vi "Full Icon Size.vi"(8 "error in":errorcluster, 11 "VI in":refnum<vi>) -> (0 "error out":errorcluster, 3 "Full Icon Size?":bool)   [LabVIEW 2024]
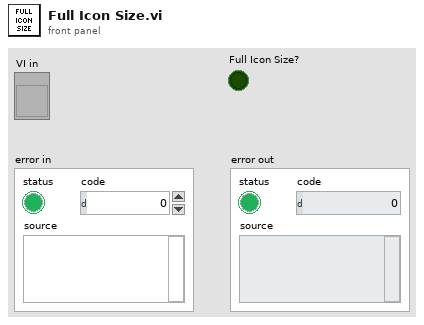
[diagram p1: front panel]
types:
  T1 = enum32{"invalid VI type", "Standard VI", "Control VI", "Global VI", "Polymorphic VI", "Configuration VI", "SubSystem", "Facade VI", "Method VI", "Statechart Diagram VI"}
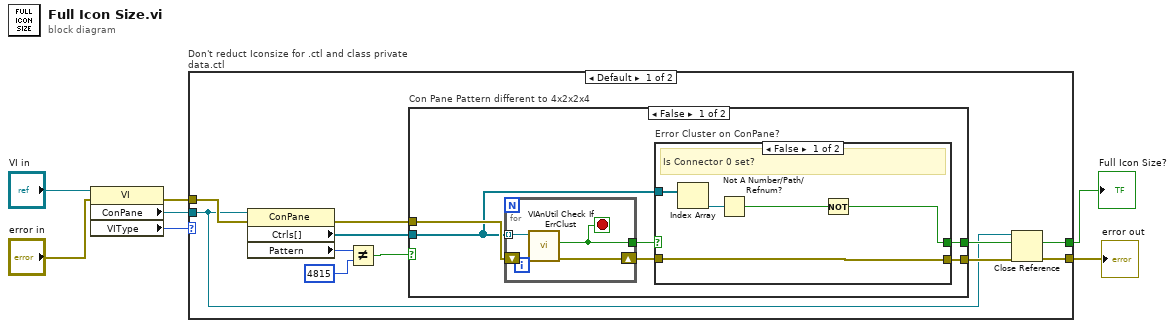
[diagram p0: block diagram]
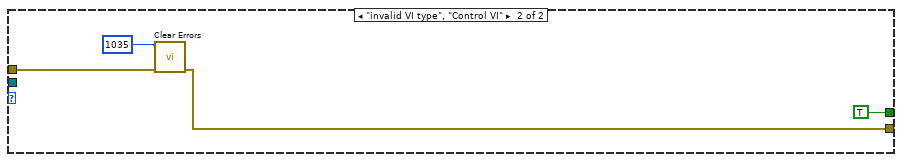
[diagram p4: hidden frame]
diagram:
  n1 = property class="VI"(reference="VI in", error in="error in") -> (error out=w5:errorcluster, "ConPane"=w2:refnum<vi>, "VIType"=w6:T1)  [unwired: 1 out]
  n2 = case "Don't reduct Iconsize for .ctl and class private data.ctl" shown="Default" w6 {
    tunnel: w2 -> [w8 _]
    tunnel: [w11 TRUE] -> w4
    tunnel: w5 -> [w17 w39]
    tunnel: [w9 w37] -> w1
    frame Default {
      n3 = property class="ConPane"(reference=w8, error in=w17) -> (error out=w16:errorcluster, "Ctrls[]"=w15:refnum<vi>[], "Pattern"=w14:u32)  [unwired: 1 out]
      n4 = Not Equal?(x=w14, y=u32 4815) -> (x != y?=w12:bool)
      n5 = case "Con Pane Pattern different to 4x2x2x4" shown="False" w12 {
        selector: w12 -> [_ w36]
        tunnel: w16 -> [w23 w35]
        tunnel: [w18 w35] -> w10
        tunnel: w15 -> [w21 _]
        tunnel: [w19 w36] -> w11
        frame False {
          n6 = for {
            tunnel: w21 -> [w34] mode=indexing
            shift-right: [w33] -> w20
            shift-left: w23 -> [w32]
            tunnel: [w31] -> w22
            stop <- w31 stop-if-true
            n7 = call <vilib>:"VIAnUtil Check If ErrClust.vi"("error in (no error)"=w32, "Control in"=w34) -> ("error out"=w33:errorcluster, "Is error cluster?"=w31:bool)  [unwired: 7 in, 1 out]
          }
          n8 = case "Error Cluster on ConPane?" shown="False" w22 {
            selector: w22 -> [_ w29]
            tunnel: w21 -> [w28 _]
            tunnel: w20 -> [w27 w30]
            tunnel: [w24 w29] -> w19
            tunnel: [w27 w30] -> w18
            frame False {
              # "Is Connector 0 set?"
              n9 = Index Array(array=w28) -> (element=w26:refnum<vi>)  [unwired: 1 in]
              n10 = Not A Number/Path/Refnum?(number/path/refnum=w26) -> (NaN/Path/Refnum?=w25:bool)
              n11 = Not(x=w25) -> (.not. x?=w24:bool)
            }
            frame True {
            }
          }
        }
        frame True {
        }
      }
      n12 = Close Reference(reference=w8, error in (no error)=w10) -> (error out=w9:errorcluster)
    }
    frame "invalid VI type", "Control VI" {
      n13 = call <vilib>:"Clear Errors.vi"("error in (no error)"=w39, "specific error code to clear (0: all)"=1035) -> ("error out"=w37:errorcluster)  [unwired: 4 in, 1 out]
    }
  }
  "Full Icon Size?" <- w4
  "error out" <- w1
